vi "叶绿素a_设置用户校准参数.vi"(8 "error in (no error)":errorcluster caption="错误输入（无错误）", 10 "用户校准参数":cluster{"K":sgl, "B":sgl}, 11 "MB_Serial session in":refnum<class "MB_Master_Serial.lvclass">) -> (0 "error out":errorcluster caption="错误输出", 3 "MB_Serial session out":refnum<class "MB_Master_Serial.lvclass">)   [LabVIEW 2016, in "斯坦道多参数.lvlib"]
uses:
  <vilib>/Plasmionique/MB Master/MB_Master_Serial/MB_Master_Serial.lvclass
  C:/Program Files (x86)/National Instruments/LabVIEW 2016/vi.lib/Plasmionique/MB Master/MB_Master/MB_Master.lvclass
  <vilib>/Plasmionique/MB Master/MB Master.lvlib
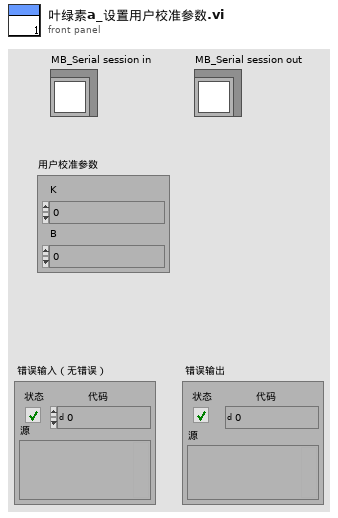
[diagram p1: front panel]
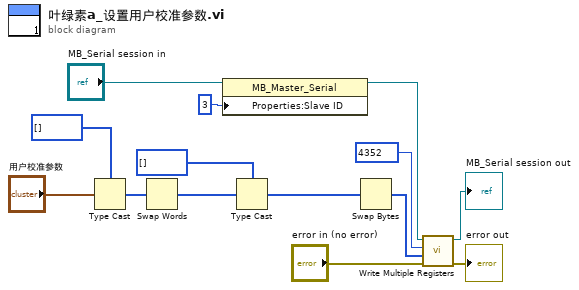
[diagram p0: block diagram]
diagram:
  n1 = Type Cast(type=u32[] [] ("数组 2"), x="用户校准参数") -> (*(type *) &x=w1:u32[])
  n2 = Swap Words(1:w1) -> (0:w6:u32[])
  n3 = property class="MB_Master_Serial"(reference="MB_Serial session in", "Properties:Slave ID"=u8 3 ("Slave ID")) -> (reference out=w9:refnum<class "MB_Master_Serial.lvclass">)  [unwired: 1 in, 1 out]
  n4 = Type Cast(type=u16[] [] ("数组 2"), x=w6) -> (*(type *) &x=w5:u16[])
  n5 = Swap Bytes(anything=w5) -> (byte swapped=w3:u16[])
  n6 = call <vilib>:"Write Multiple Registers.vi"("error in (no error)"="error in (no error)", "values"=w3, "starting address"=u16 4352, "MB session in"=w9) -> ("error out"=→"error out":errorcluster, "MB session out"=→"MB_Serial session out":refnum<class "MB_Master_Serial.lvclass">)  [unwired: 6 in]
